vi "Self Event Alias.vi"(11 "eeeee in":refnum<class "eeeee.lvclass">) -> (2 "Self Event Alias":string)   [LabVIEW 2021, in "Providers.lvlib" / "eeeee.lvlib" / "eeeee.lvclass"]
uses:
  eeeee.lvclass
  eeeee.lvclass/eeeee.ctl
  jettl/Event/Event.lvclass
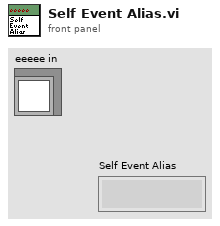
[diagram p1: front panel]
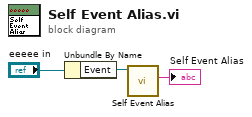
[diagram p0: block diagram]
diagram:
  n1 = Unbundle By Name("eeeee in") -> ("Event"=w2:refnum<class "Event.lvclass">)
  n2 = call-dynamic "Self Event Alias.vi"("Event in"=w2) -> ("Self Event Alias"=→"Self Event Alias":string)  [unwired: 10 in]
